vi "Get_QR_Image.vi"(6 "strEncodeData":string="yinpei", 7 "nMaskingNo":i32, 8 "error in (no error)":errorcluster caption="错误输入（无错误）", 9 "bAutoExtent":i32, 10 "nVersion":i32, 11 "nLevel":i32) -> (0 "error out":errorcluster caption="错误输出", 1 "p_nVersion":i32, 2 "p_buf":i8[](array[numeric]), 3 "p_len_m":i32)   [LabVIEW 2016, in "QR_ENCODE.lvlib"]
doc: "QR_ENCODE_API void GetImage(int nLevel, int nVersion, BOOL bAutoExtent, int nMaskingNo, LPCSTR strEncodeData,int *p_len_m,BYTE *p_buf,int *p_nVersion) ;\n\nQR_ENCODE_API void GetImage(int nLevel, int nVersion, BOOL bAutoExtent, int nMaskingNo,char *strEncodeData,int *p_len_m,BYTE *p_buf,int *p_nVersion) ;"
uses:
  QR_ENCODE.lvlib
  QR_ENCODE.dll
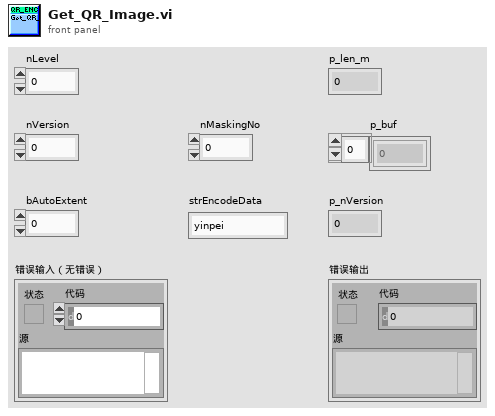
[diagram p1: front panel]
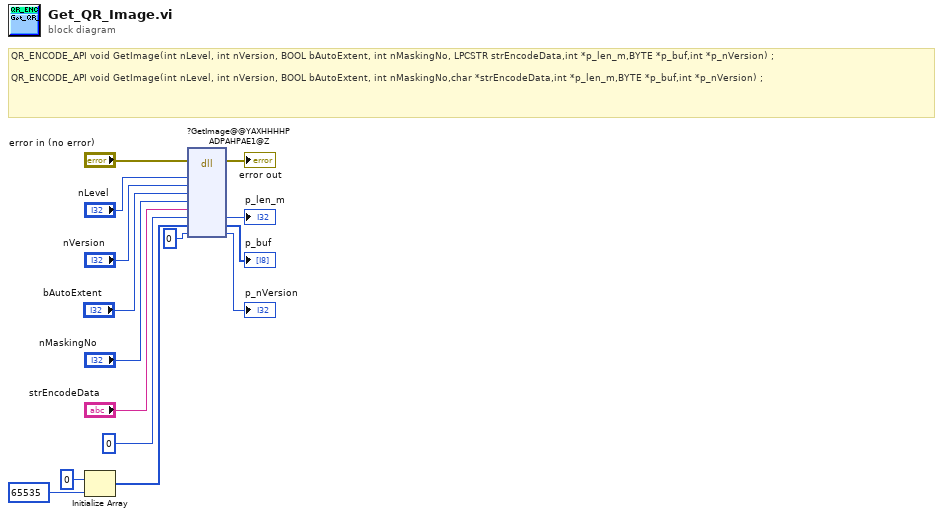
[diagram p0: block diagram]
diagram:
  # "QR_ENCODE_API void GetImage(int nLevel, int nVersion, BOOL bAutoExtent, int nMaskingNo, LPCSTR strEncodeData,int *p_len_m,BYTE *p_buf,int *p_nVersion) ;\n\nQR_ENCODE_API void GetImage(int nLevel, int nVersion, BOOL bAutoExtent, int nMaskingNo,char *strEncodeData,int *p_len_m,BYTE *p_buf,int *p_nVersion) ;"
  n1 = Initialize Array(i8 0 ("元素"), 65535 ("维数大小")) -> (w8:i8[])
  n2 = dll-call lib="PTH2abs F\tgitkrakenéææ¨¡æ¿!ä¸ä½ç«é¡¹ç®æ ·æ¿ï¼æ¨¡æ¿ï¼ä¸ä½ç«é¡¹ç® - V4è´¨æ§APIOpSignInAPI\tQR_ENCODEQR_ENCODE.*" fn="?GetImage@@YAXHHHHPADPAHPAE1@Z"(error in="error in (no error)", "nLevel"="nLevel", "nVersion"="nVersion", "bAutoExtent"="bAutoExtent", "nMaskingNo"="nMaskingNo", "strEncodeData"="strEncodeData", "p_len_m"=0, "p_buf"=w8, "p_nVersion"=0) -> (error out=→"error out":errorcluster, "p_len_m"=→"p_len_m":i32, "p_buf"=→"p_buf":i8[], "p_nVersion"=→"p_nVersion":i32)  [unwired: 8 in, 1 out]
